vi "LVCAM Destroy Self.vi"(11 "LVCAM Destroy Self Msg in":refnum<class "LVCAM Destroy Self Msg.lvclass">) -> (0 "error out":errorcluster, 1 "Destroyed Self?":bool, 3 "LVCAM Destroy Self Msg out":refnum<class "LVCAM Destroy Self Msg.lvclass">)   [LabVIEW 2021, in "LVCAM Destroy Self.lvlib" / "LVCAM Destroy Self Msg.lvclass"]
uses:
  LVCAM Destroy Self Msg.lvclass
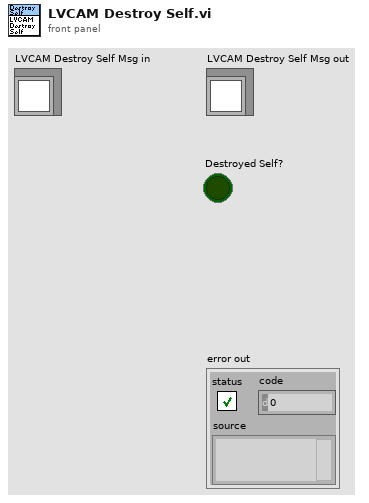
[diagram p1: front panel]
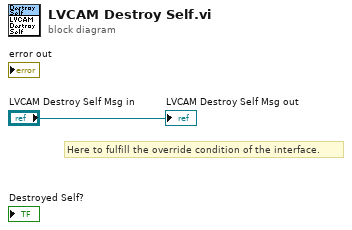
[diagram p0: block diagram]
diagram:
  # "Here to fulfill the override condition of the interface."
  "LVCAM Destroy Self Msg out" <- "LVCAM Destroy Self Msg in"
